vi "Multi Data Processor No Objects.vi"(8 "error in (no error)":errorcluster, 11 "Synapse CCD in":T4={"JYCCDLib.IJYCCDReqd"=refnum, "JYMONOLib.IJYMonoReqd"=refnum, "Integration time"=0.01, "ADC"=0, "GAIN"=0, "Areas"=[[1, 1, 1, 1024, 256, 1, 256]], "Most Recent Data Object"=refnum, "Mono Properties"={"Grating"=0, "Center Wavelength"=0.0, "Entrance Slit"=0.0, "Exit Slit"=0.0}, "Coverage"={"Max"=0.0, "Min"=0.0}, "Multi-Acquisitions"={"Dark Subtract?"=FALSE, "Averaging?"=FALSE, "Cosmic Ray Removal?"=FALSE, "# to Average"=0, "Time Between Acq."=0, "Acquisitions Control Array"=[TRUE], "Raw Data"=[], "Processed Data"=[], "Array of Wavelengths"=[]}, "Channel Names"=[], "Channel Units"=[]} {"ADC" items=["   20 kHz", "1 MHz", "1 MHz Ultra"]; "GAIN" items=["High Light", "Best Dynamic", "High Sensitivity"]; "Mono Properties"."Grating" items=["1200 lines/mm - 500 nm Blaze", "1200 lines/mm - 750 nm Blaze", "600 lines/mm - 1000 nm Blaze"]}) -> (0 "error out":errorcluster, 1 "Processed Array":dbl[](array[numeric]), 2 "Processed Spectrum":cluster{"Ramp Pattern":dbl[], "X array":dbl[]}[](graph), 3 "Synapse CCD out":T4={"JYCCDLib.IJYCCDReqd"=refnum, "JYMONOLib.IJYMonoReqd"=refnum, "Integration time"=0.01, "ADC"=0, "GAIN"=0, "Areas"=[[1, 1, 1, 1024, 256, 1, 256]], "Most Recent Data Object"=refnum, "Mono Properties"={"Grating"=0, "Center Wavelength"=0.0, "Entrance Slit"=0.0, "Exit Slit"=0.0}, "Coverage"={"Max"=0.0, "Min"=0.0}, "Multi-Acquisitions"={"Dark Subtract?"=FALSE, "Averaging?"=FALSE, "Cosmic Ray Removal?"=FALSE, "# to Average"=0, "Time Between Acq."=0, "Acquisitions Control Array"=[TRUE], "Raw Data"=[], "Processed Data"=[], "Array of Wavelengths"=[]}, "Channel Names"=[], "Channel Units"=[]} {"ADC" items=["   20 kHz", "1 MHz", "1 MHz Ultra"]; "GAIN" items=["High Light", "Best Dynamic", "High Sensitivity"]; "Mono Properties"."Grating" items=["1200 lines/mm - 500 nm Blaze", "1200 lines/mm - 750 nm Blaze", "600 lines/mm - 1000 nm Blaze"]})   [LabVIEW 2009]
doc: "Processes Multi-Data based on member data Booleans. Returns Single Spectrum Plot and stores data in member data.\n\nPossible options include:\n\nDark Subtraction\nAveraging Multiple Scans\nCosmic Ray Removal"
uses:
  Areas.ctl
  Utility Classes/Readable/Channel Names.ctl
  Utility Classes/Readable/Channel Units.ctl
  Synapse CCD.lvclass
  Utility Classes/Readable/Readable.lvclass
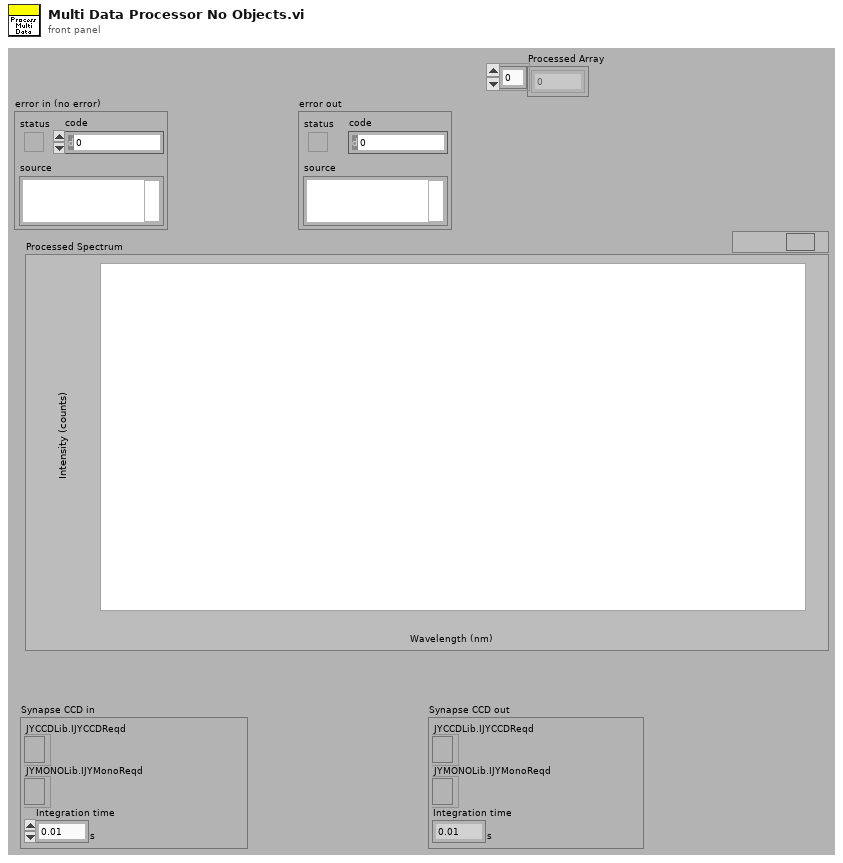
[diagram p1: front panel]
types:
  T1 = typedef "Synapse CCD.lvclass/Areas.ctl" = i32[][]
  T2 = typedef "Readable.lvclass/Channel Names.ctl" = string[]
  T3 = typedef "Readable.lvclass/Channel Units.ctl" = string[]
  T4 = cluster{"JYCCDLib.IJYCCDReqd":refnum<k7>, "JYMONOLib.IJYMonoReqd":refnum<k7>, "Integration time":dbl[unit], "ADC":u16, "GAIN":u16, "Areas":T1, "Most Recent Data Object":refnum<k7>, "Mono Properties":cluster{"Grating":u16, "Center Wavelength":dbl[unit], "Entrance Slit":dbl[unit], "Exit Slit":dbl[unit]}, "Coverage":cluster{"Max":dbl[unit], "Min":dbl[unit]}, "Multi-Acquisitions":cluster{"Dark Subtract?":bool, "Averaging?":bool, "Cosmic Ray Removal?":bool, "# to Average":u32, "Time Between Acq.":u32, "Acquisitions Control Array":bool[], "Raw Data":i32[][], "Processed Data":dbl[], "Array of Wavelengths":dbl[]}, "Channel Names":T2, "Channel Units":T3}
  T5 = cluster{"Array of Wavelengths":dbl[], "Processed Data":dbl[]}
  T6 = cluster{"Array of Wavelengths":dbl[], "Processed Data":dbl[]}[]
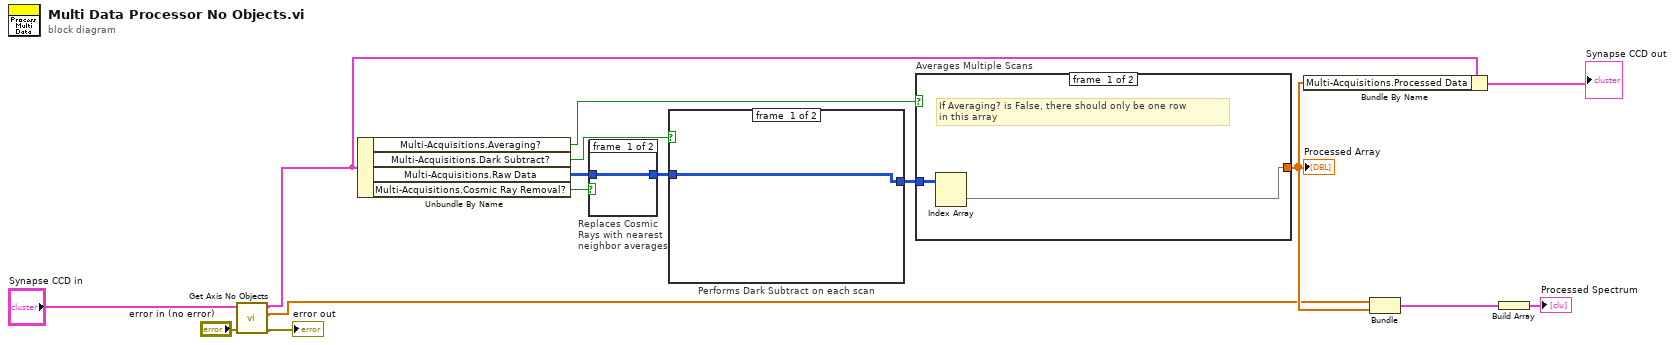
[diagram p0: block diagram]
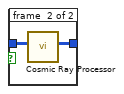
[diagram p2: hidden frame]
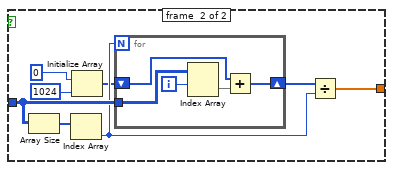
[diagram p3: hidden frame]
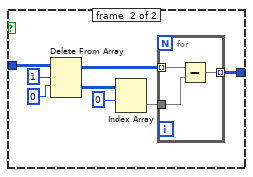
[diagram p4: hidden frame]
diagram:
  n1 = call "Get Axis No Objects.vi"("error in (no error)"="error in (no error)", "Synapse CCD in"="Synapse CCD in") -> ("error out"=→"error out":errorcluster, "Array of Wavelengths"=w3:dbl[], "Synapse CCD out"=w4:T4)  [unwired: 7 in]
  n2 = Unbundle By Name(w4) -> ("Multi-Acquisitions.Averaging?"=w13:bool, "Multi-Acquisitions.Dark Subtract?"=w14:bool, "Multi-Acquisitions.Raw Data"=w8:i32[][], "Multi-Acquisitions.Cosmic Ray Removal?"=w9:bool)
  n3 = case "Replaces Cosmic\nRays with nearest\nneighbor averages" shown="True" w9 {
    tunnel: w8 -> [w16 w18]
    tunnel: [w16 w17] -> w7
    frame #0 {
    }
    frame #1 {
      n4 = call "Cosmic Ray Processor.vi"("Raw Data"=w18) -> ("Processed Data"=w17:i32[][])  [unwired: 10 in]
    }
  }
  n5 = case "Performs Dark Subtract on each scan" shown="True" w14 {
    tunnel: w7 -> [w19 w24]
    tunnel: [w19 w21] -> w15
    frame #0 {
    }
    frame #1 {
      n6 = Delete From Array(array=w24, length=1, index (row)=0) -> (deleted portion=w20:i32[][], array with subset deleted=w25:i32[][])  [unwired: 1 in]
      n7 = Index Array(array=w20, index (row)=0) -> (element=w22:i32[])  [unwired: 1 in]
      n8 = for {
        tunnel: w25 -> [w30] mode=indexing
        tunnel: w22 -> [w29]
        tunnel: [w28] -> w21 mode=indexing
        n9 = Subtract(x=w30, y=w29) -> (x-y=w28:i32[])
      }
    }
  }
  n10 = case "Averages Multiple Scans" shown="True" w13 {
    tunnel: w15 -> [w32 w39]
    tunnel: [w31 w36] -> w10
    frame #0 {
      # "If Averaging? is False, there should only be one row\nin this array"
      n11 = Index Array(array=w32) -> (element=w31:i32[])  [unwired: 2 in]
    }
    frame #1 {
      n12 = Array Size(array=w39) -> (size(s)=w40:i32[])
      n13 = Index Array(array=w40) -> (element=w37:i32)  [unwired: 1 in]
      n14 = Initialize Array(0, 1024) -> (w33:i32[])
      n15 = for {
        N: w37 -> [_]
        tunnel: w39 -> [w43]
        shift-right: [w41] -> w38
        shift-left: w33 -> [w45]
        i -> [w44]
        n16 = Index Array(array=w43, index (row)=w44) -> (element=w42:i32[])  [unwired: 1 in]
        n17 = Add(x=w45, y=w42) -> (x+y=w41:i32[])
      }
      n18 = Divide(x=w38, y=w37) -> (x/y=w36:dbl[])
    }
  }
  "Processed Array" <- w10
  n19 = Bundle By Name(cluster=w4, "Multi-Acquisitions.Processed Data"=w10) -> (→"Synapse CCD out":T4)
  n20 = Bundle("Array of Wavelengths"=w3, "Processed Data"=w10) -> (w12:T5)  [unwired: 1 in]
  n21 = Build Array(w12) -> (→"Processed Spectrum":T6)
